vi "Waveform Loop.vi"(8 "error in (no error)":errorcluster, 11 "Message Queues out":T1) -> (0 "error out":errorcluster)   [LabVIEW 2018, in "Waveform Loop.lvlib"]
uses:
  Waveform Loop.lvlib
  Main/Main Queue Cluster.ctl
  support/Message Queue/Message Cluster.ctl
  Waveform Loop State Cluster.ctl
  <vilib>/Platform/TimedLoop/XDataNode/timing_clust.ctl
  <vilib>/Platform/TimedLoop/XDataNode/nitl_modes.ctl
  <vilib>/Platform/TimedLoop/XDataNode/wakeup.ctl
  Start Params Cluster.ctl
  support/Message Queue/Enqueue Message (Single).vi
  Main/Main Globals.vi
  <vilib>/Platform/TimedLoop/XDataNode/XDataNode.xnode
  <vilib>/Platform/TimedLoop/XDataNode/XDNodeRunTimeDep.lvlib
  support/Message Queue/Message Queue.lvlib
  support/Command Log VIs/Command Logging.lvlib
panel:
  out "i":i32
  out "dt":i64
  out "Actual Start [i]":i64
  out "dt (seconds)":dbl
  in  "Latch Samples":bool
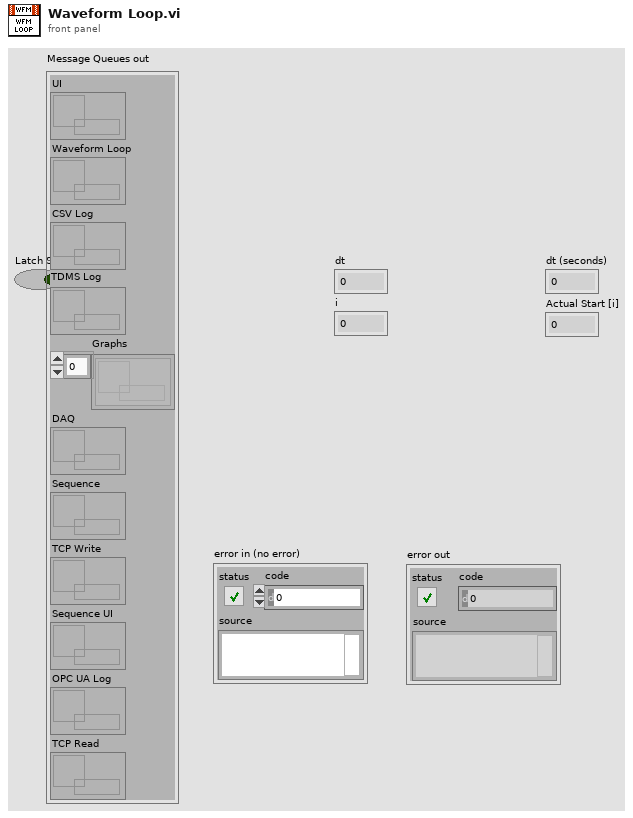
[diagram p1: front panel]
types:
  T1 = typedef "Main Queue Cluster.ctl" = cluster{"UI":refnum<queue>, "Waveform Loop":refnum<queue>, "CSV Log":refnum<queue>, "TDMS Log":refnum<queue>, "Graphs":refnum<queue>[], "DAQ":refnum<queue>, "Sequence":refnum<queue>, "TCP Write":refnum<queue>, "Sequence UI":refnum<queue>, "OPC UA Log":refnum<queue>, "TCP Read":refnum<queue>}
  T2 = typedef "Waveform Loop.lvlib/Waveform Loop State Cluster.ctl" = cluster{"Waveform template":waveform(dbl)}
  T3 = typedef "XDNodeRunTimeDep.lvlib/timing_clust.ctl" = cluster{"Expected End [f-1]":u64, "Actual End [f-1]":u64, "Finished Late? [f-1]":bool, "Expected End [i-1]":u64, "Actual End [i-1]":u64, "Finished Late? [i-1]":bool, "Expected Start [i]":u64, "Actual Start [i]":u64, "Expected Start [f]":u64, "Actual Start [f]":u64, "Source Name":string, "Structure Name":string, "Period":i64, "Deadline":i64, "Offset":i64, "Start":i64, "Priority":i32, "Timeout":i32, "Mode":T4, "Wakeup Reason":T5, "Error":errorcluster, "Source Type":string, "Secondary Source Type":string, "Global End Time":u64, "Global Start Time":u64, "Frame Duration":u64, "Iteration Duration":u64, "Assigned CPU":i32, "I/O Scan Engine Mode":u32}
  T4 = typedef "XDNodeRunTimeDep.lvlib/nitl_modes.ctl" = enum32{"No Change", "Process missed periods, maintain original phase", "Discard missed periods, maintain original phase", "Process missed periods, ignore original phase", "Discard missed periods, ignore original phase"}
  T5 = typedef "XDNodeRunTimeDep.lvlib/wakeup.ctl" = enum32{"Normal", "Aborted", "Asynchronous wakeup", "Timing source error", "Timed loop error", "Timeout"}
  T6 = typedef "Waveform Loop.lvlib/Start Params Cluster.ctl" = cluster{"dt (seconds)":dbl, "CSV Logfile path":path, "TDMS Logfile path":path}
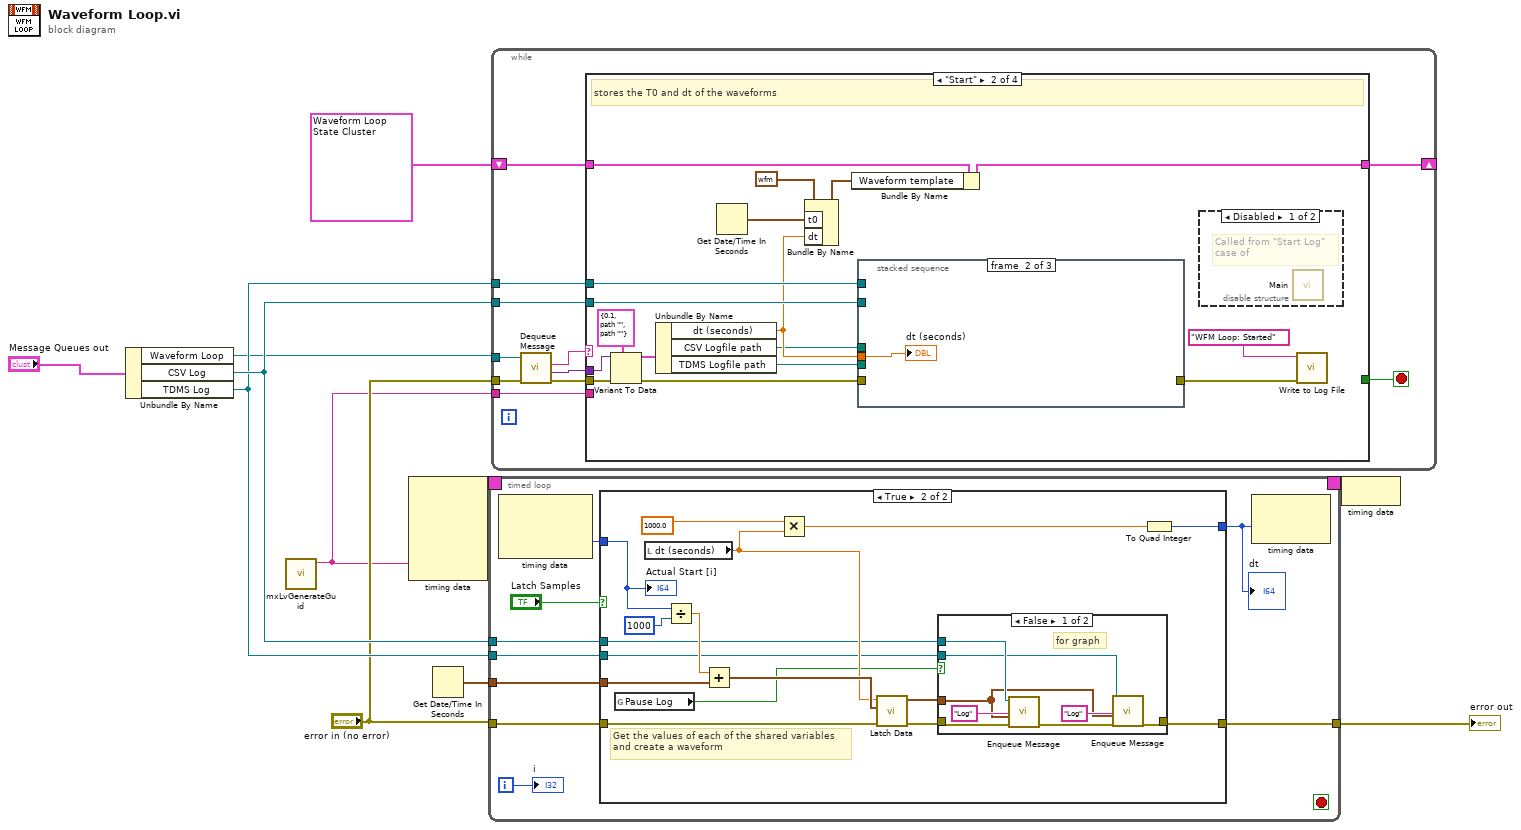
[diagram p0: block diagram]
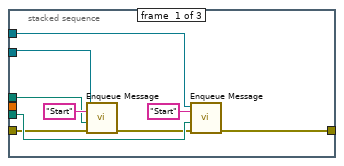
[diagram p4: hidden frame]
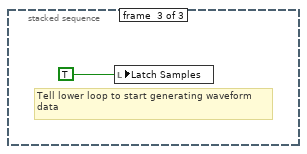
[diagram p5: hidden frame]
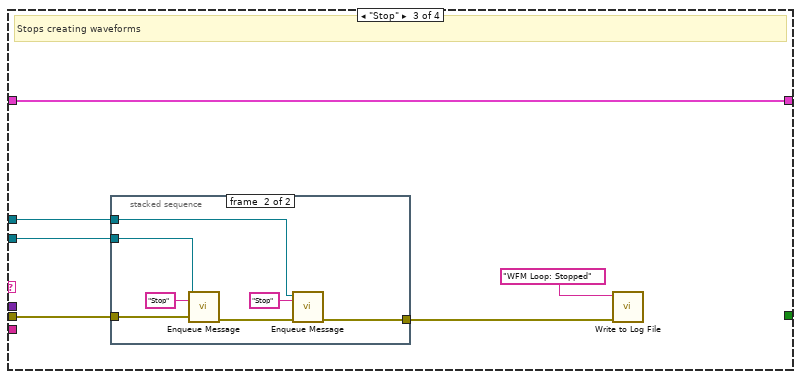
[diagram p6: hidden frame]
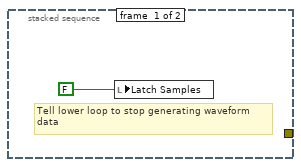
[diagram p7: hidden frame]
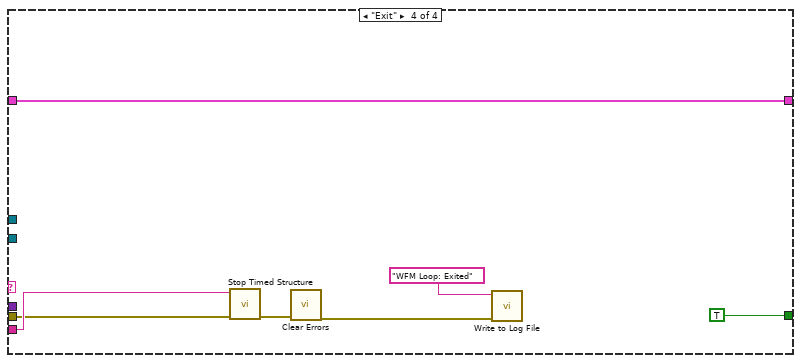
[diagram p8: hidden frame]
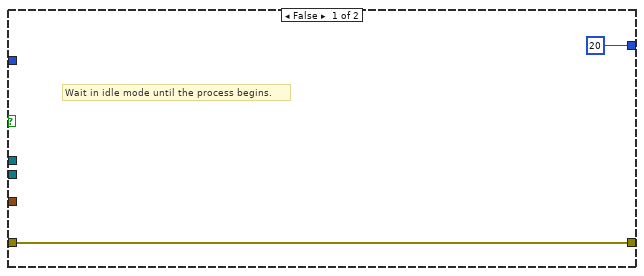
[diagram p9: hidden frame]
diagram:
  n1 = Unbundle By Name("Message Queues out") -> ("Waveform Loop"=w4:refnum<queue>, "CSV Log"=w6:refnum<queue>, "TDMS Log"=w5:refnum<queue>)
  n2 = call <resource>:"mxLvGenerateGuid.vi"() -> ("Value"=w1:string)  [unwired: 10 in, 1 out]
  n3 = node-c288(w1) -> (w11:T3)  [unwired: 4 in]
  n4 = Get Date/Time In Seconds() -> (seconds since 1Jan1904=w7:timestamp)
  n5 = timed-loop {
    timing: w11 -> [_]
    timing-out: [_] -> w10
    tunnel: w7 -> [w18]
    tunnel: "error in (no error)" -> [w17]
    tunnel: w6 -> [w16]
    tunnel: w5 -> [w15]
    tunnel: [w14] -> w3
    i -> [w13]
    stop <- _ stop-if-true
    n6 = node-c288() -> (w19:i64)  [unwired: 1 in, 2 out]
    n7 = case shown="True" "Latch Samples" {
      tunnel: [i64 20 w37] -> w12
      tunnel: w19 -> [_ w36]
      tunnel: w18 -> [_ w33]
      tunnel: w17 -> [w21 w31]
      tunnel: [w21 w26] -> w14
      tunnel: w16 -> [_ w28]
      tunnel: w15 -> [_ w27]
      frame False {
        # "Wait in idle mode until the process begins."
      }
      frame True {
        # "Get the values of each of the shared variables\nand create a waveform"
        n8 = global read "Main Globals.vi" "Pause Log"() -> (w23:bool)
        n9 = local read "dt (seconds)"() -> (w29:dbl)
        n10 = Divide(x=w36, y=i64 1000) -> (x/y=w34:dbl)
        n11 = Add(x=w34, y=w33) -> (x+y=w32:timestamp)
        n12 = Multiply(x=1000.0 ("y"), y=w29) -> (x*y=w38:dbl)
        n13 = call "Latch Data.vi"("error in (no error)"=w31, "Time Stamp"=w32, "dt"=w29) -> ("error out"=w24:errorcluster, "Waveform Array"=w25:waveform(dbl)[])  [unwired: 7 in]
        n14 = case shown="False" w23 {
          tunnel: w28 -> [w46 _]
          tunnel: w27 -> [w45 _]
          tunnel: [w44 w47] -> w26
          tunnel: w25 -> [w41 _]
          tunnel: w24 -> [w40 w47]
          frame False {
            # "for graph"
            n15 = call-poly "Enqueue Message.vi"("error in (no error)"=w40, "Message Data"=w41, "Message"="Log", "Message Queue"=w46) -> ("error out"=w39:errorcluster)  [unwired: 6 in, 1 out]
            n16 = call-poly "Enqueue Message.vi"("error in (no error)"=w39, "Message Data"=w41, "Message"="Log", "Message Queue"=w45) -> ("error out"=w44:errorcluster)  [unwired: 6 in, 1 out]
          }
          frame True {
          }
        }
        n17 = To Quad Integer(1:w38) -> (0:w37:i64)
        "Actual Start [i]" <- w36
      }
    }
    "dt" <- w12
    n18 = node-c288(w12) -> ()  [unwired: 1 in, 1 out]
    "i" <- w13
  }
  "error out" <- w3
  n19 = while {
    shift-right: [w60] -> _
    shift-left: T2 {"Waveform template"={"t0"=timestamp(0 s since 1904-01-01), "dt"=1.0, "Y"=[]}} ("Waveform Loop State") -> [w62]
    tunnel: w6 -> [w58]
    tunnel: w5 -> [w59]
    tunnel: w4 -> [w55]
    tunnel: "error in (no error)" -> [w54]
    tunnel: w1 -> [w53]
    stop <- w56 stop-if-true
    n20 = call "Dequeue Message.vi"("error in (no error)"=w54, "Message Queue"=w55) -> ("error out"=w57:errorcluster, "Message Data"=w61:variant, "Message"=w63:string)  [unwired: 6 in, 1 out]
    n21 = case shown="\"Start\"" w63 {
      tunnel: w62 -> [w64 w81 w95 w113]
      tunnel: w61 -> [_ w78 _ _]
      tunnel: [w64 w77 w95 w113] -> w60
      tunnel: w59 -> [_ w76 w98 _]
      tunnel: w58 -> [_ w75 w97 _]
      tunnel: w57 -> [_ w68 w96 w109]
      tunnel: [_ _ _ TRUE] -> w56
      tunnel: w53 -> [_ _ _ w111]
      frame Default {
        # "This case should not be called"
      }
      frame "Start" {
        # "stores the T0 and dt of the waveforms"
        n22 = Variant To Data(error in=w68, type=T6 {"dt (seconds)"=0.1, "CSV Logfile path"=path "", "TDMS Logfile path"=path ""} ("Start Params"), Variant=w78) -> (data=w72:T6, error out=w67:errorcluster)
        n23 = Unbundle By Name(w72) -> ("dt (seconds)"=w71:dbl, "CSV Logfile path"=w70:path, "TDMS Logfile path"=w69:path)
        n24 = Get Date/Time In Seconds() -> (seconds since 1Jan1904=w80:timestamp)
        n25 = Bundle By Name(cluster=waveform(dbl) {"t0"=timestamp(0 s since 1904-01-01), "dt"=1.0, "Y"=[]} ("Waveform template"), "t0"=w80, "dt"=w71) -> (w79:waveform(dbl))
        n26 = Bundle By Name(cluster=w81, "Waveform template"=w79) -> (w77:T2)
        n27 = stacked-sequence {
          tunnel: w71 -> [_ w91 _]
          tunnel: w76 -> [w89 _ _]
          tunnel: w75 -> [w87 _ _]
          tunnel: w70 -> [w86 _ _]
          tunnel: w69 -> [w85 _ _]
          tunnel: w67 -> [w84 _ _]
          tunnel: [w82 _ _] -> w65
          frame #0 {
            n28 = call-poly "Enqueue Message.vi"("error in (no error)"=w84, "Message Data"=w86, "Message"="Start", "Message Queue"=w87) -> ("error out"=w83:errorcluster)  [unwired: 6 in, 1 out]
            n29 = call-poly "Enqueue Message.vi"("error in (no error)"=w83, "Message Data"=w85, "Message"="Start", "Message Queue"=w89) -> ("error out"=w82:errorcluster)  [unwired: 6 in, 1 out]
          }
          frame #1 {
            "dt (seconds)" <- w91
          }
          frame #2 {
            # "Tell lower loop to start generating waveform\ndata"
            n30 = local write "Latch Samples"(TRUE ("Latch Samples")) -> ()
          }
        }
        n31 = disable-structure shown="Disabled" {
          frame Disabled {
            # "Called from \"Start Log\"\ncase of"
            n32 = call "Main.vi"() -> ()  [unwired: 12 in]
          }
          frame Enabled {
          }
        }
        n33 = call "Write to Log File.vi"("error in"=w65, "text"="WFM Loop: Started") -> ()  [unwired: 9 in, 1 out]
      }
      frame "Stop" {
        # "Stops creating waveforms"
        n34 = stacked-sequence {
          tunnel: w98 -> [_ w105]
          tunnel: w97 -> [_ w103]
          tunnel: w96 -> [_ w102]
          tunnel: [_ w100] -> w93
          frame #0 {
            # "Tell lower loop to stop generating waveform\ndata"
            n35 = local write "Latch Samples"(FALSE ("Latch Samples")) -> ()
          }
          frame #1 {
            n36 = call-poly "Enqueue Message.vi"("error in (no error)"=w102, "Message"="Stop", "Message Queue"=w103) -> ("error out"=w101:errorcluster)  [unwired: 7 in, 1 out]
            n37 = call-poly "Enqueue Message.vi"("error in (no error)"=w101, "Message"="Stop", "Message Queue"=w105) -> ("error out"=w100:errorcluster)  [unwired: 7 in, 1 out]
          }
        }
        n38 = call "Write to Log File.vi"("error in"=w93, "text"="WFM Loop: Stopped") -> ()  [unwired: 9 in, 1 out]
      }
      frame "Exit" {
        n39 = call <vilib>:"Stop Timed Structure.vi"("error in (no error)"=w109, "name"=w111) -> ("error out"=w110:errorcluster)  [unwired: 9 in]
        n40 = call <vilib>:"Clear Errors.vi"("error in (no error)"=w110) -> ("error out"=w107:errorcluster)  [unwired: 5 in, 1 out]
        n41 = call "Write to Log File.vi"("error in"=w107, "text"="WFM Loop: Exited") -> ()  [unwired: 9 in, 1 out]
      }
    }
  }
  n42 = node-c288(w10) -> ()
